vi "FTW-Endpoint-ConnectToListener.vi"(0 "FTW-Endpoint In":refnum<class "FTW-Endpoint-TCP.lvclass">, 5 "Address":string, 9 "Timeout":i32=1000 format="%dmsec", 11 "error in":errorcluster) -> (4 "FTW-Endpoint Out":refnum<class "FTW-Endpoint-TCP.lvclass">, 6 "Actual Address":string, 15 "error out":errorcluster)   [LabVIEW 2015, in "FTW-Endpoint-TCP.lvclass"]
uses:
  FTW-Endpoint-TCP.lvclass
  FTW-Endpoint-TCP.lvclass/FTW-Endpoint-TCP.ctl
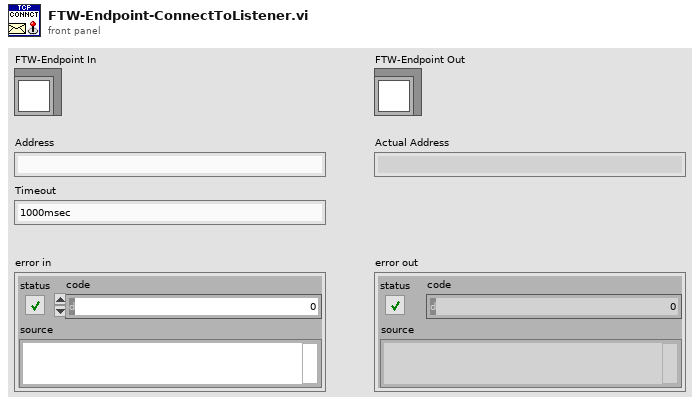
[diagram p1: front panel]
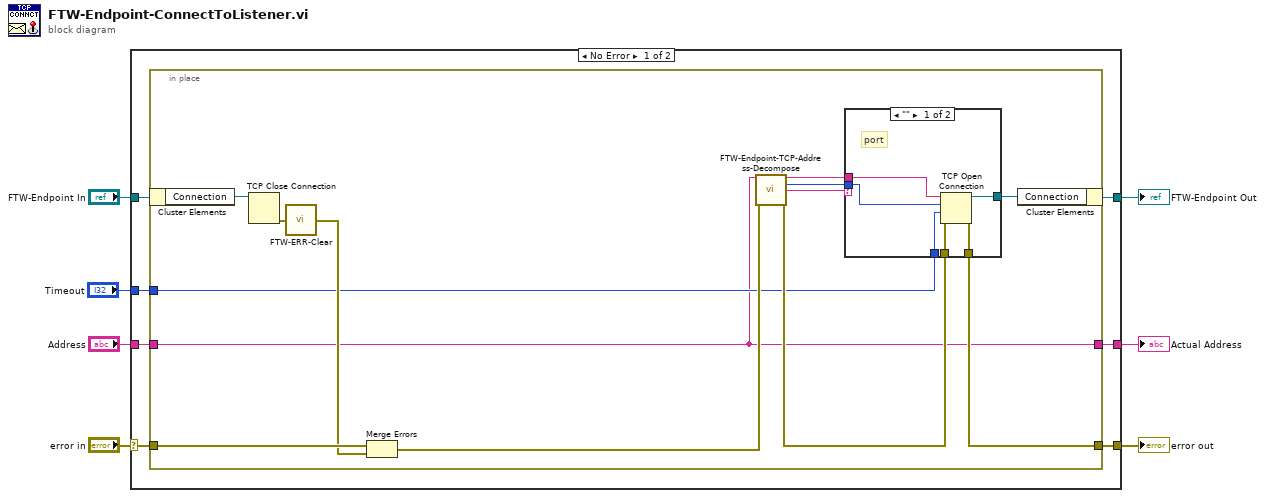
[diagram p0: block diagram]
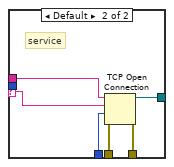
[diagram p2: hidden frame]
diagram:
  n1 = case shown="No Error" "error in" {
    selector: "error in" -> [w14 w41]
    tunnel: [w13 w41] -> w7
    tunnel: [w12 w40] -> w6
    tunnel: "FTW-Endpoint In" -> [w11 w40]
    tunnel: "Address" -> [w10 _]
    tunnel: [w9 _] -> w2
    tunnel: "Timeout" -> [w8 _]
    frame No Error {
      n2 = in-place {
        in-place-border: w14 -> [w23]
        in-place-border: [w24] -> w13
        in-place-border: w10 -> [w18]
        in-place-border: [w18] -> w9
        in-place-border: w8 -> [w19]
        n3 = in-place-cluster #1(w11) -> ("Connection"=w27:refnum<k5>)
        n4 = TCP Close Connection(connection ID=w27) -> (error out=w26:errorcluster)  [unwired: 2 in, 1 out]
        n5 = call "FTW-ERR-Clear.vi"("error to snuff"=w26) -> ("no error"=w20:errorcluster)
        n6 = Merge Errors(w23, w20) -> (w21:errorcluster)
        n7 = call "FTW-Endpoint-TCP-Address-Decompose.vi"("Endpoint Address"=w18, "error in"=w21) -> ("Domain"=w17:string, "Port"=w15:u16, "Service Name"=w16:string, "error out"=w22:errorcluster)  [unwired: 10 in]
        n8 = case shown="\"\"" w16 {
          selector: w16 -> [_ w34]
          tunnel: w15 -> [w28 _]
          tunnel: [w33 w39] -> w25
          tunnel: [w32 w38] -> w24
          tunnel: w17 -> [w29 w37]
          tunnel: w22 -> [w31 w36]
          tunnel: w19 -> [w30 w35]
          frame "" {
            # "port"
            n9 = TCP Open Connection(address=w29, remote port or service name=w28, timeout ms (60000)=w30, error in (no error)=w31) -> (connection ID=w33:refnum<k5>, error out=w32:errorcluster)  [unwired: 1 in]
          }
          frame Default {
            # "service"
            n10 = TCP Open Connection(address=w37, remote port or service name=w34, timeout ms (60000)=w35, error in (no error)=w36) -> (connection ID=w39:refnum<k5>, error out=w38:errorcluster)  [unwired: 1 in]
          }
        }
        n11 = in-place-cluster #1("Connection"=w25) -> (w12:refnum<class "FTW-Endpoint-TCP.lvclass">)
      }
    }
    frame Error {
    }
  }
  "FTW-Endpoint Out" <- w6
  "error out" <- w7
  "Actual Address" <- w2
